vi "Align Elements.vi"(6 "Variant in":variant, 7 "Shift Pressed?":bool, 8 "error in (no error)":errorcluster, 10 "QD Combo Box Ref":refnum<vi>, 11 "QD Launch VI Ref":refnum<vi>) -> (0 "error out":errorcluster, 4 "Variant out":variant)   [LabVIEW 2016, in "Align Elements.lvlib"]
doc: "Align and distribute elements of a selection.\n\nUsage:\nSelect some elements on the frontpanel or the blockdiagram.\nPress Ctrl+Space Ctrl+A to open a small UI with alignment buttons next to the current mouse pointer position.\n\nIf a button is pressed the selection of elements will be aligned or distributed to the wanted choice.\nThe panel can be closed using the window's close button or by pressing the ESC key.\n\nIt is also possible to align the elements with the WASD keys\nW...Top\nS...Bottom\nA...Left\nD...Right\nC...Horizontal Center\nV...Vertical Center\n\nQ...Vertical Gap\nE...Horizontal Gap\n\nIf the alignment is controlled by the keys the panel will immediatelly be closed.\n\nThe plugin provides better results for the alignment by hiding the increment/decrement buttons of numeric controls during the execution.\n\nDefault Shortcut - [A]"
uses:
  _Align Elements/Align Elements.lvlib
panel:
  # "Do not change the connector pane of this VI.\n\nSee the block diagram for directions on how to use this template."
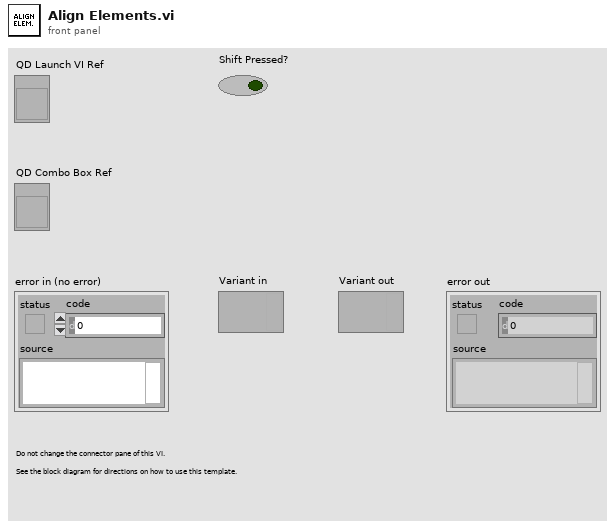
[diagram p1: front panel]
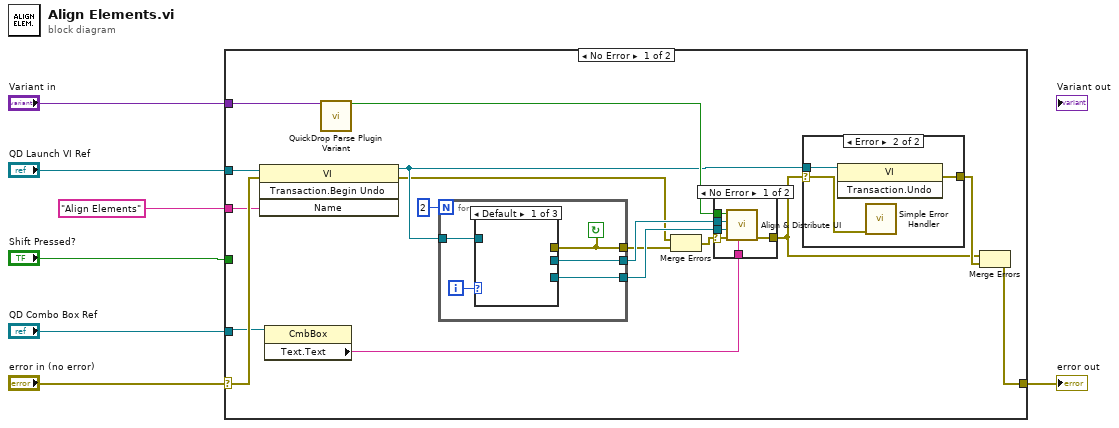
[diagram p0: block diagram]
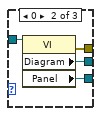
[diagram p2: hidden frame]
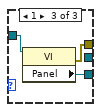
[diagram p3: hidden frame]
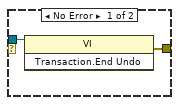
[diagram p5: hidden frame]
diagram:
  n1 = case shown="No Error" "error in (no error)" {
    selector: "error in (no error)" -> [w23 w49]
    tunnel: [w14 w49] -> w1
    tunnel: "Variant in" -> [w24 _]
    tunnel: "QD Launch VI Ref" -> [w21 _]
    tunnel: "Align Elements" ("Undo Name") -> [w22 _]
    tunnel: "Shift Pressed?" -> [_ _]
    tunnel: "QD Combo Box Ref" -> [w16 _]
    frame No Error {
      n2 = invoke class="VI" method="Transaction.Begin Undo"(reference=w21, error in=w23, "Name"=w22) -> (reference out=w12:refnum<vi>, error out=w9:errorcluster)  [unwired: 1 in, 2 out]
      n3 = property class="CmbBox"(reference=w16) -> ("Text.Text"=w15:string)  [unwired: 1 in, 2 out]
      n4 = call <vilib>:"QuickDrop Parse Plugin Variant.vi"("QDKS Variant in"=w24) -> ("QD Launch VI Panel?"=w19:bool)  [unwired: 12 in, 2 out]
      n5 = for {
        N: 2 -> [_]
        tunnel: [w29] -> w18
        tunnel: [w28] -> w17
        tunnel: w12 -> [w27]
        tunnel: [w25] -> w8
        i -> [w26]
        stop <- w25 continue-if-true
        n6 = case shown="Default" w26 {
          tunnel: [_ w33 _] -> w29
          tunnel: [_ w32 w36] -> w28
          tunnel: w27 -> [_ w31 w35]
          tunnel: [_ w30 w34] -> w25
          frame Default {
          }
          frame 0 {
            n7 = property class="VI"(reference=w31) -> (error out=w30:errorcluster, "Diagram"=w33:refnum<vi>, "Panel"=w32:refnum<vi>)  [unwired: 1 in, 1 out]
          }
          frame 1 {
            n8 = property class="VI"(reference=w35) -> (error out=w34:errorcluster, "Panel"=w36:refnum<vi>)  [unwired: 1 in, 1 out]
          }
        }
      }
      n9 = Merge Errors(w9, w8) -> (w10:errorcluster)
      n10 = case shown="No Error" w10 {
        selector: w10 -> [w39 w43]
        tunnel: w19 -> [w42 _]
        tunnel: w18 -> [w41 _]
        tunnel: w17 -> [w40 _]
        tunnel: w15 -> [w38 _]
        tunnel: [w37 w43] -> w13
        frame No Error {
          n11 = call "Align & Distribute UI.vi"("Predefined Input Key"=w38, "error in (no error)"=w39, "Panel Ref"=w40, "Block Diagram Ref"=w41, "Executed on Frontpanel?"=w42) -> ("error out"=w37:errorcluster)  [unwired: 4 in, 2 out]
        }
        frame Error {
        }
      }
      n12 = case shown="Error" w13 {
        selector: w13 -> [_ w46]
        tunnel: [w45 w48] -> w20
        tunnel: w12 -> [w44 w47]
        frame No Error {
          n13 = invoke class="VI" method="Transaction.End Undo"(reference=w44) -> (error out=w45:errorcluster)  [unwired: 2 in, 2 out]
        }
        frame Error {
          n14 = invoke class="VI" method="Transaction.Undo"(reference=w47) -> (error out=w48:errorcluster)  [unwired: 2 in, 2 out]
          n15 = call <vilib>:"Simple Error Handler.vi"("error in (no error)"=w46) -> ()  [unwired: 4 in, 5 out]
        }
      }
      n16 = Merge Errors(w13, w20) -> (w14:errorcluster)
    }
    frame Error {
    }
  }
  "error out" <- w1
